vi "Util Multiline String to Array.vi"(7 "delimiter (LF)":string, 8 "error in (no error)":errorcluster, 11 "String Input":string) -> (0 "error out":errorcluster, 3 "Line Array":string[](array[string]))   [LabVIEW 2017, in "xHelper.lvlib"]
uses:
  xHelper.lvlib
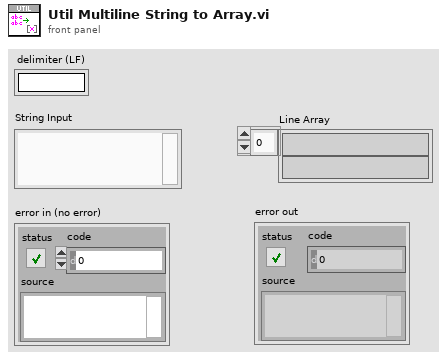
[diagram p1: front panel]
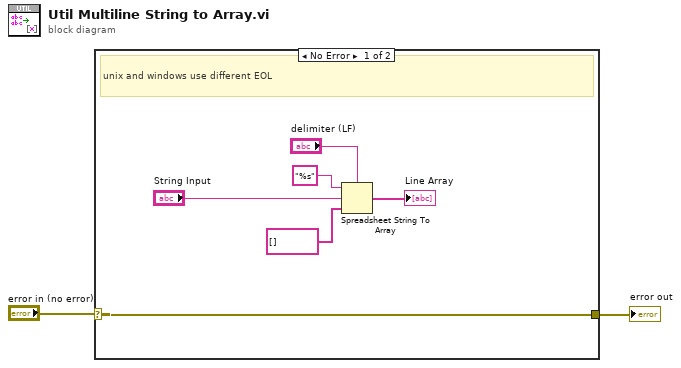
[diagram p0: block diagram]
diagram:
  n1 = case shown="No Error" "error in (no error)" {
    selector: "error in (no error)" -> [w4 w9]
    tunnel: [w4 w9] -> w1
    frame No Error {
      # "unix and windows use different EOL"
      n2 = Spreadsheet String To Array(delimiter (Tab)="delimiter (LF)", format string="%s", spreadsheet string="String Input", array type (2D Dbl)=string[] []) -> (array=→"Line Array":string[])
    }
    frame Error {
    }
  }
  "error out" <- w1
